vi "2-Arithmetic&Logic Calculator.vi"() -> ()   [LabVIEW 2020]
panel:
  in  "x1-decimal":i32
  in  "x-decimal":i32
  out "Result-Binary":i32 format="%08b"
  in  "Calculate":bool
  out "x-binary":i32 format="%08b"
  in  "Function selector":T1(ring)
  out "Result-Decimal":i32
  out "x1-binary":i32 format="%08b"
  in  "stop":bool
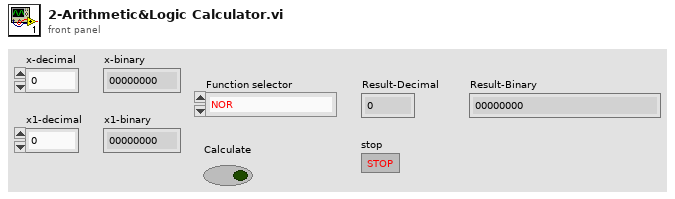
[diagram p1: front panel]
types:
  T1 = enum16{"NOR", "ADDITION", "MULTIPLICATION", "XOR", "OR", "AND", "SUBTRACTION"}
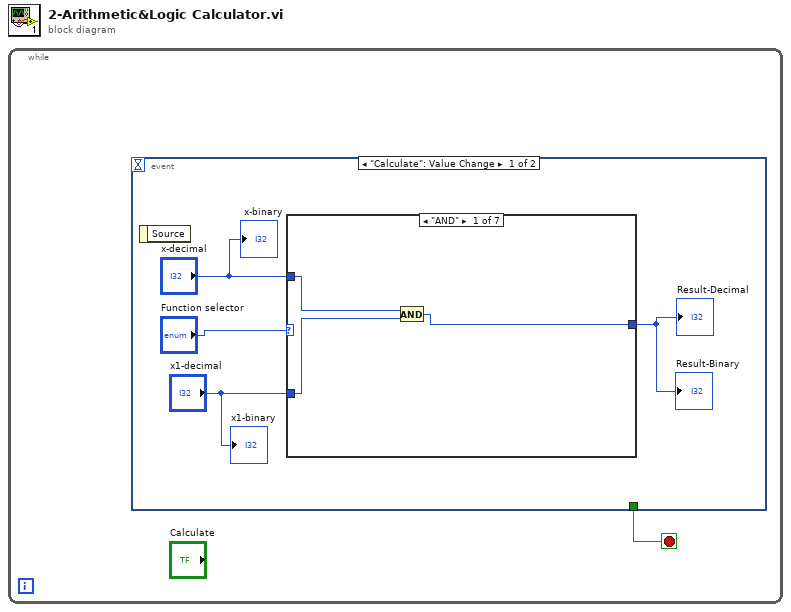
[diagram p0: block diagram]
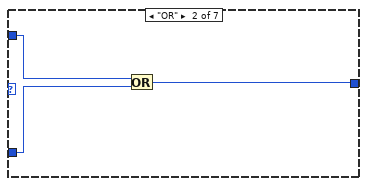
[diagram p2: hidden frame]
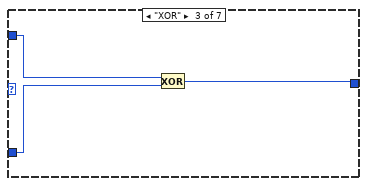
[diagram p3: hidden frame]
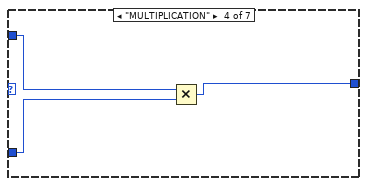
[diagram p4: hidden frame]
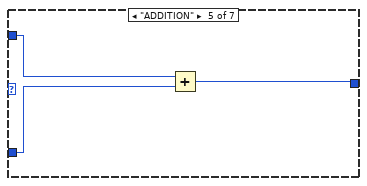
[diagram p5: hidden frame]
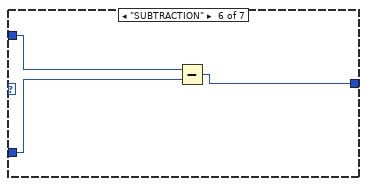
[diagram p6: hidden frame]
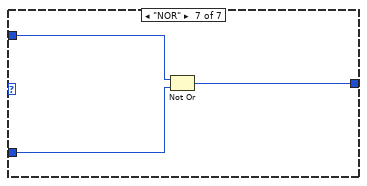
[diagram p7: hidden frame]
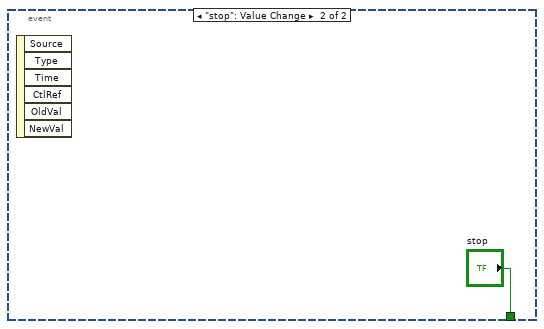
[diagram p8: hidden frame]
diagram:
  n1 = while {
    stop <- w1 stop-if-true
    n2 = event shown="[0] \"Calculate\": Value Change" {
      selector: _ -> [_ _]
      dyn-events: _ -> [_ _]
      timeout: _ -> [_ _]
      tunnel: [_ "stop"] -> w1
      event "Calculate": Value Change {
        n3 = event-data() -> ()  [unwired: 1 in, 1 out]
        n4 = case shown="\"AND\"" "Function selector" {
          tunnel: "x-decimal" -> [w8 w11 w13 w17 w20 w23 w26]
          tunnel: "x1-decimal" -> [w7 w10 w14 w16 w19 w22 w25]
          tunnel: [w6 w9 w12 w15 w18 w21 w24] -> w2
          frame "AND" {
            n5 = And(x=w8, y=w7) -> (x .and. y?=w6:i32)
          }
          frame "OR" {
            n6 = Or(x=w11, y=w10) -> (x .or. y?=w9:i32)
          }
          frame "XOR" {
            n7 = Exclusive Or(1:w14, 2:w13) -> (0:w12:i32)
          }
          frame "MULTIPLICATION" {
            n8 = Multiply(x=w17, y=w16) -> (x*y=w15:i32)
          }
          frame "ADDITION" {
            n9 = Add(x=w20, y=w19) -> (x+y=w18:i32)
          }
          frame "SUBTRACTION" {
            n10 = Subtract(x=w23, y=w22) -> (x-y=w21:i32)
          }
          frame "NOR" {
            n11 = Not Or(1:w25, 2:w26) -> (0:w24:i32)
          }
        }
        "Result-Decimal" <- w2
        "Result-Binary" <- w2
        "x-binary" <- "x-decimal"
        "x1-binary" <- "x1-decimal"
      }
      event "stop": Value Change {
        n12 = event-data() -> ()  [unwired: 1 in, 6 out]
      }
    }
  }
